vi "Get Section Text.vi"(10 "Section Name":string, 11 "Data":string) -> (1 "Section Found?":bool, 2 "Section Text":string)   [LabVIEW 2020, in "MGI Path Selector.lvclass"]
doc: "Extract the text for the specified section.\n\nAuthored by Shawn Walpole\nsupport@mooregoodideas.com\nwww.mooregoodideas.com\n\nCopyright (c) 2013, Moore Good Ideas, Inc.\n\nAll rights reserved.\n\nRedistribution and use in source and binary forms, with or without modification, are permitted provided that the following conditions are met:\n\n * Redistributions of source code must retain the above copyright notice, this list of conditions and the following disclaimer.\n * Redistributions in binary form must reproduce the above copyright notice, this list of conditions and the following disclaimer in the documentation and/or other materials provided with the distribution.\n * Neither the name of Moore Good Ideas, Inc. nor the names of its contributors may be used to endorse or promote products derived from this software without specific prior written permission.\n\nTHIS SOFTWARE IS PROVIDED BY THE COPYRIGHT HOLDERS AND CONTRIBUTORS \"AS IS\" AND ANY EXPRESS OR IMPLIED WARRANTIES, INCLUDING, BUT NOT LIMITED TO, THE IMPLIED WARRANTIES OF MERCHANTABILITY AND FITNESS FOR A PARTICULAR PURPOSE ARE DISCLAIMED. IN NO EVENT SHALL THE COPYRIGHT OWNER OR CONTRIBUTORS BE LIABLE FOR ANY DIRECT, INDIRECT, INCIDENTAL, SPECIAL, EXEMPLARY, OR CONSEQUENTIAL DAMAGES (INCLUDING, BUT NOT LIMITED TO, PROCUREMENT OF SUBSTITUTE GOODS OR SERVICES; LOSS OF USE, DATA, OR PROFITS; OR BUSINESS INTERRUPTION) HOWEVER CAUSED AND ON ANY THEORY OF LIABILITY, WHETHER IN CONTRACT, STRICT LIABILITY, OR TORT (INCLUDING NEGLIGENCE OR OTHERWISE) ARISING IN ANY WAY OUT OF THE USE OF THIS SOFTWARE, EVEN IF ADVISED OF THE POSSIBILITY OF SUCH DAMAGE."
uses:
  <userlib>/_MGI/User Interface/Path Selector XControl/Class Hierarchy/MGI Path Selector.lvclass
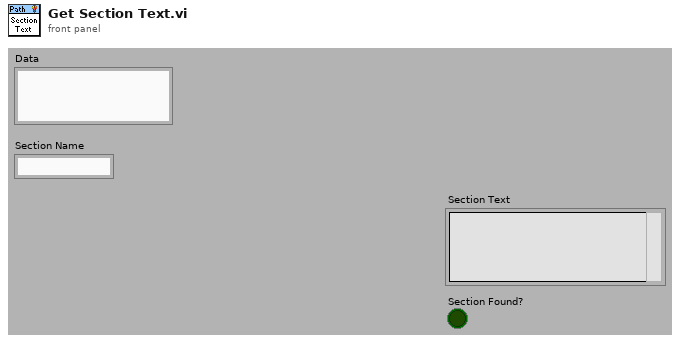
[diagram p1: front panel]
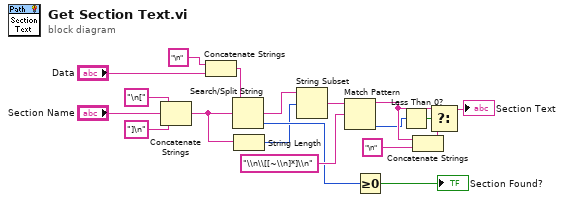
[diagram p0: block diagram]
diagram:
  n1 = Concatenate Strings("\n[" ("string"), "Section Name", "]\n" ("string")) -> (w13:string)
  n2 = Concatenate Strings("\n" ("string"), "Data") -> (w15:string)
  n3 = Search/Split String(string=w15, search string/char (-)=w13) -> (match + rest of string=w1:string, offset of match=w16:i32)  [unwired: 1 in, 1 out]
  n4 = String Length(string=w13) -> (length=w12:i32)
  n5 = String Subset(string=w1, offset (0)=w12) -> (substring=w14:string)  [unwired: 1 in]
  n6 = Match Pattern(string=w14, regular expression="\\n\\[[~\\n]*]\\n") -> (before substring=w9:string, offset past match=w7:i32)  [unwired: 3 out]
  n7 = Greater Or Equal To 0?(x=w16) -> (x >= 0?=→"Section Found?":bool)
  n8 = Less Than 0?(x=w7) -> (x < 0?=w6:bool)
  n9 = Concatenate Strings(w9, "\n" ("string")) -> (w10:string)
  n10 = Select(t=w9, s=w6, f=w10) -> (s? t:f=→"Section Text":string)
